vi "CheckUnknown.vi"(6 "Status":refnum<vi>, 8 "error in (no error)":errorcluster, 9 "Known Found?":bool, 10 "filenames":string[](array[string]), 11 "Working Dir":path) -> (0 "error out":errorcluster, 1 "Abort?":bool, 3 "Working Dir Out":path)   [LabVIEW 2022 SP3]
uses:
  TypeDefs/Tag Cmd.ctl
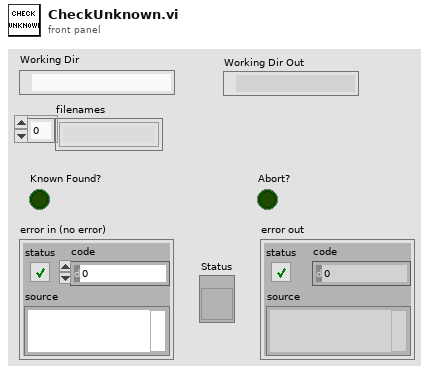
[diagram p1: front panel]
types:
  T1 = typedef "Tag Cmd.ctl" = enum16{"Init", "Get Known", "Set Known"}
  T2 = enum16{"Left Button", "Center Button", "Right Button", "Window Close"}
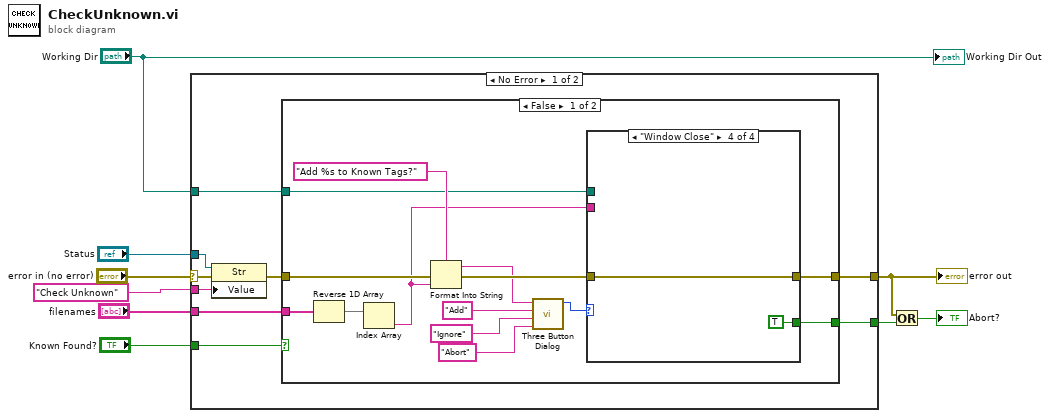
[diagram p0: block diagram]
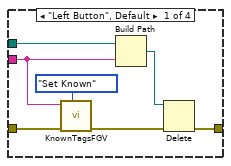
[diagram p2: hidden frame]
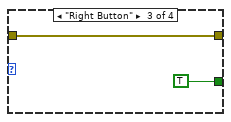
[diagram p4: hidden frame]
diagram:
  n1 = case shown="No Error" "error in (no error)" {
    selector: "error in (no error)" -> [w10 w46]
    tunnel: "Known Found?" -> [w18 _]
    tunnel: [w17 w46] -> w2
    tunnel: "filenames" -> [w16 _]
    tunnel: "Working Dir" -> [w15 _]
    tunnel: "Status" -> [w13 _]
    tunnel: "Check Unknown" ("Value") -> [w12 _]
    tunnel: [w11 _] -> w3
    frame No Error {
      n2 = property class="Str"(reference=w13, error in=w10, "Value"=w12) -> (error out=w14:errorcluster)  [unwired: 1 out]
      n3 = case shown="False" w18 {
        tunnel: [w25 w45] -> w17
        tunnel: w14 -> [w30 w45]
        tunnel: w15 -> [w27 _]
        tunnel: w16 -> [w32 _]
        tunnel: [w19 _] -> w11
        frame False {
          n4 = Reverse 1D Array(array=w32) -> (reversed array=w31:string[])
          n5 = Index Array(array=w31) -> (element=w26:string)  [unwired: 1 in]
          n6 = Format Into String(format string="Add %s to Known Tags?", error in=w30, w26) -> (resulting string=w21:string, error out=w28:errorcluster)  [unwired: 1 in]
          n7 = call <vilib>:"Three Button Dialog.vi"("Right Button Text (\"Cancel\")"="Abort" ("Right Button Text (\"Cancel\")"), "Center Button Text (\"No\")"="Ignore" ("F button name (\"Cancel\")"), "Left Button Text (\"Yes\")"="Add" ("T button name (\"OK\")"), "message"=w21) -> ("Which Button?"=w20:T2)  [unwired: 7 in]
          n8 = case shown="\"Window Close\"" w20 {
            tunnel: w28 -> [w37 w40 w42 w43]
            tunnel: w27 -> [w39 _ _ _]
            tunnel: w26 -> [w34 _ _ _]
            tunnel: [w33 w40 w42 w43] -> w25
            tunnel: [_ _ TRUE TRUE] -> w19
            frame "Left Button", Default {
              n9 = call "KnownTagsFGV.vi"("Tag Cmd"=Tag_Cmd."Set Known", "error in (no error)"=w37, "New Tag"=w34) -> ("error out"=w36:errorcluster)  [unwired: 7 in, 1 out]
              n10 = Build Path(base path=w39, name or relative path=w34) -> (appended path=w38:path)
              n11 = Delete(path (use dialog)=w38, error in=w36) -> (error out=w33:errorcluster)  [unwired: 3 in, 2 out]
            }
            frame "Center Button" {
            }
            frame "Right Button" {
            }
            frame "Window Close" {
            }
          }
        }
        frame True {
        }
      }
    }
    frame Error {
    }
  }
  "error out" <- w2
  n12 = Or(x=w2, y=w3) -> (x .or. y?=→"Abort?":bool)
  "Working Dir Out" <- "Working Dir"
